vi "Kinect Create.vi"(11 "Depth Format":i32(ring)=1 items=["Undefined", "Resolution640x480Fps30", "Resolution320x240Fps30", "Resolution80x60Fps30"]) -> (0 "error out":errorcluster, 3 "Kinect Acquisition Queue":refnum<queue>)   [LabVIEW 2011]
uses:
  Kinect Data Cluster.ctl
  Microsoft.Kinect
  Kinect Global Status.vi
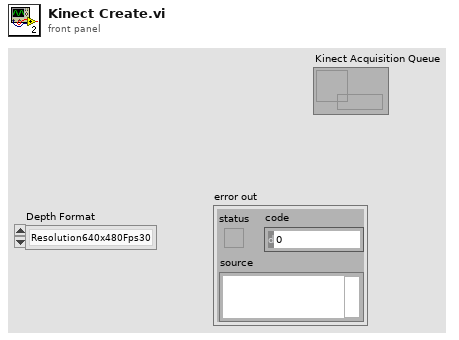
[diagram p1: front panel]
types:
  T1 = typedef "Kinect Data Cluster.ctl" = cluster{"1D Depth Data":i16[], "Width":i32, "Height":i32, "Timestamp":i32}
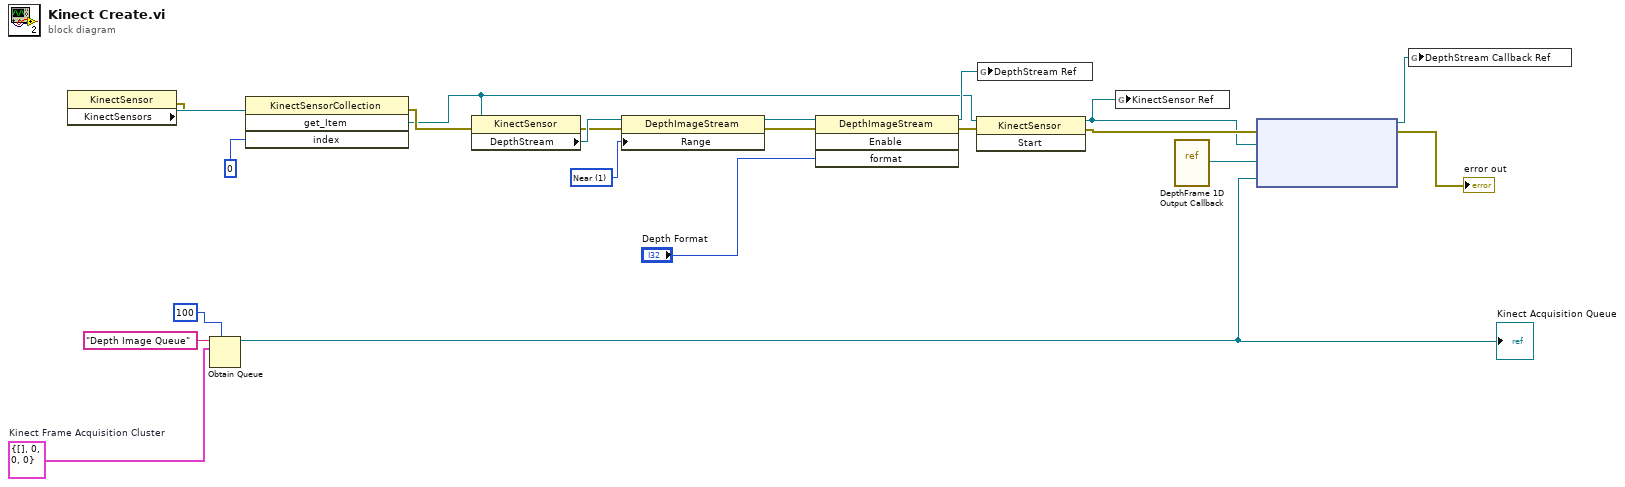
[diagram p0: block diagram]
diagram:
  w2 = T1 {"1D Depth Data"=[], "Width"=0, "Height"=0, "Timestamp"=0}  # Kinect Frame Acquisition Cluster
  w7 = 1 items=["Default", "Near"] ("Range")
  n1 = property class="KinectSensor"() -> (error out=w20:errorcluster, "KinectSensors"=w22:refnum<k24>)  [unwired: 2 in, 1 out]
  n2 = Obtain Queue(max queue size (-1, unlimited)=100, name (unnamed)="Depth Image Queue", element data type=w2) -> (queue out=w3:refnum<queue>)  [unwired: 2 in, 2 out]
  "Kinect Acquisition Queue" <- w3
  n3 = invoke class="KinectSensorCollection" method="get_Item"(reference=w22, error in=w20, "index"=0) -> (error out=w19:errorcluster, "get_Item"=w10:refnum<k24>)  [unwired: 1 in, 2 out]
  n4 = property class="KinectSensor"(reference=w10, error in=w19) -> (error out=w8:errorcluster, "DepthStream"=w9:refnum<k24>)  [unwired: 1 out]
  n5 = property class="DepthImageStream"(reference=w9, error in=w8, "Range"=w7) -> (reference out=w6:refnum<k24>, error out=w5:errorcluster)
  n6 = invoke class="DepthImageStream" method="Enable"(reference=w6, error in=w5, "format"="Depth Format") -> (reference out=w15:refnum<k24>, error out=w18:errorcluster)  [unwired: 1 in, 2 out]
  n7 = invoke class="KinectSensor" method="Start"(reference=w10, error in=w18) -> (reference out=w14:refnum<k24>, error out=w17:errorcluster)  [unwired: 1 in, 1 out]
  n8 = global write "Kinect Global Status.vi" "DepthStream Ref"(w15) -> ()
  n9 = global write "Kinect Global Status.vi" "KinectSensor Ref"(w14) -> ()
  n10 = vi-ref "DepthFrame 1D Output Callback.vi"() -> (w1:refnum<vi>)
  n11 = node(w17, w14, w1, w3) -> (w13:refnum<k27>, →"error out":errorcluster)  [unwired: 1 in]
  n12 = global write "Kinect Global Status.vi" "DepthStream Callback Ref"(w13) -> ()
